vi "Speed Estimation (1 Motor with IC).vi"(0 "waveforms":waveform(dbl)[](array[waveform]), 1 "fundamental frequency [Hz]":dbl=50.0, 2 "reset? (F)":bool, 7 "speed estimation settings":cluster{"% overlap":dbl, "algorithm":T2}={"% overlap"=0.0, "algorithm"=enum."3-phase signals"}, 9 "initial conditions":T1 {"zoom FFT settings"."FFT settings"."window" items=["Rectangle"=0, "Hanning"=1, "Hamming"=2, "Blackman-Harris"=3, "Exact Blackman"=4, "Blackman"=5, "Flat Top"=6, "4 Term B-Harris "=7, "7 Term B-Harris"=8, "Low Sidelobe"=9, "Blackman Nuttall"=11, "Triangle"=30, "Bartlett-Hanning"=31, "Bohman"=32, "Parzen"=33, "Welch"=34, "Kaiser"=60, "Dolph-Chebyshev"=61, "Gaussian"=62]}, 11 "error in (no error)":errorcluster, 12 "nameplate information":T4, 13 "window length (60 s)":dbl=60.0) -> (3 "new data available?":bool, 4 "speed [RPM]":dbl, 6 "slip":dbl, 10 "final conditions":T1 {"zoom FFT settings"."FFT settings"."window" items=["Rectangle"=0, "Hanning"=1, "Hamming"=2, "Blackman-Harris"=3, "Exact Blackman"=4, "Blackman"=5, "Flat Top"=6, "4 Term B-Harris "=7, "7 Term B-Harris"=8, "Low Sidelobe"=9, "Blackman Nuttall"=11, "Triangle"=30, "Bartlett-Hanning"=31, "Bohman"=32, "Parzen"=33, "Welch"=34, "Kaiser"=60, "Dolph-Chebyshev"=61, "Gaussian"=62]}, 15 "error out":errorcluster)   [LabVIEW 2014, in "NI_EP_Motor Monitoring.lvlib"]
doc: "Calculates the motor speed. You must manually select the polymorphic instance you want to use."
uses:
  <vilib>/addons/Electrical Power/Motor Monitoring/NI_EP_Motor Monitoring.lvlib
  <vilib>/addons/Electrical Power/Motor Monitoring/subVIs/ep_Demodulation Algorithm.ctl
  <vilib>/addons/Electrical Power/Motor Monitoring/subVIs/ep_Initial Conditions for Speed Estimation.ctl
  <vilib>/addons/Electrical Power/Motor Monitoring/subVIs/ep_Zoom FFT Settings.ctl
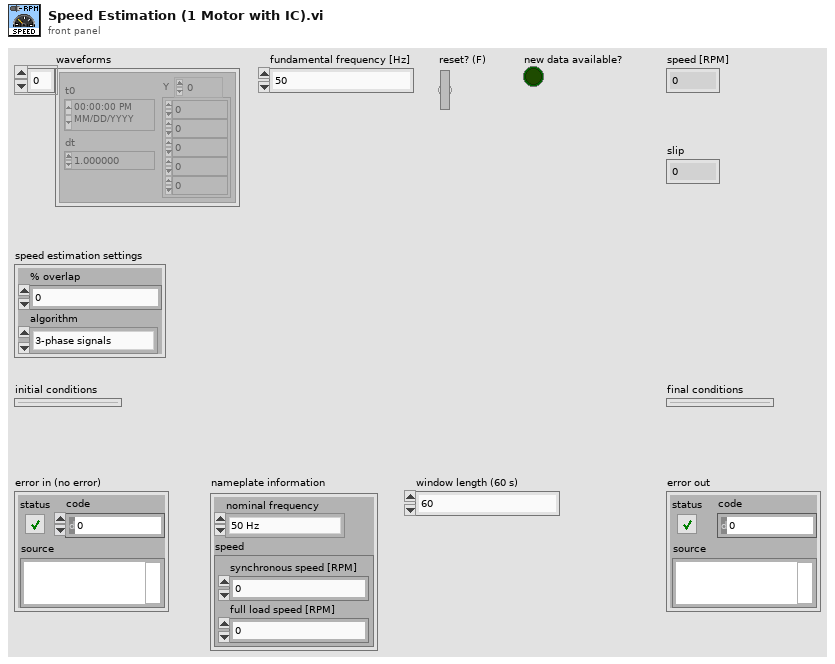
[diagram p1: front panel]
types:
  T1 = typedef "NI_EP_Motor Monitoring.lvlib/ep_Initial Conditions for Speed Estimation.ctl" = cluster{"SVAF state":cluster{"space vector amplitude":dbl, "hilbert state":cluster{"delay conditions":dbl[], "filter conditions":dbl[]}}, "zoom FFT state":cluster{"phase state":dbl, "zoom FFT state":cluster{"zoom settings state":cluster{"zoom":i32, "stop band attenuation":enum16{"84 dB", "96 dB", "120 dB"}, "alias protect in final transition":bool, "oversampling ratio":dbl}, "SML Decimation Filter (complex input) state":cluster{"decimation settings state":cluster{"M":i32, "stop band attenuation":enum16{"84 dB", "96 dB", "120 dB"}, "alias protect in transition band":bool, "oversampling ratio":dbl}, "counter for garbage samples state":i32, "sml_Parameter Setting for Zoom Factor state":cluster{"filter length * interpolation state":i32, "interpolation state":i32, "comb filter order state":i32, "CFIR par state":cluster{"h":dbl[], "M":i32, "N":i32}, "LFIR par state":cluster{"h":dbl[], "M":i32, "N":i32}, "CIC Stages state":i32}, "aal_CIC (complex input) state":cluster{"aal_cascaded moving average (complex input) state":cluster{"states":cdb[], "circular buffers state":cdb[][], "circular buffer counter state":i32}, "aal_moving average with decimation by order (complex input) state":cluster{"residue result state":cdb, "processed data counter state":i32}}, "sml_Cascaded Decimation Filter (complex input) CFIR state":cluster{"unprocessed data state":cdb[], "final conditions state":cdb[][], "sml_M-1 Decimator with IC (complex input) state":cluster{"coefficients in reverse order state":dbl[], "max index for coefficients state":i32}}, "sml_Cascaded Decimation Filter (complex input) LFIR state":cluster{"unprocessed data state":cdb[], "final conditions state":cdb[][], "sml_M-1 Decimator with IC (complex input) state":cluster{"coefficients in reverse order state":dbl[], "max index for coefficients state":i32}}}, "ma_SML Data Packing (complex input) state":cluster{"array getting packed state":cdb[], "last array processed state":cdb[], "index state":i32, "packing parameters state":cluster{i32, "size":i32}}}, "FFT{X} [Vrms]":cdb[]}, "speed state":cluster{"speed [RPM]":dbl, "slip":dbl}, "speed estimation settings":cluster{"% overlap":dbl, "algorithm":T2}, "filter information":cluster{"coefficients":dbl[], "order":i32}, "zoom FFT settings":T3, "last valid window":i32, "fund. frequency for averager":dbl[]}
  T2 = typedef "NI_EP_Motor Monitoring.lvlib/ep_Demodulation Algorithm.ctl" = enum16{"1-phase signal", "3-phase signals"}
  T3 = typedef "NI_EP_Motor Monitoring.lvlib/ep_Zoom FFT Settings.ctl" = cluster{"FFT settings":cluster{"window":u16, "Window Size":i32, "FFT Size":i32, "%overlap":dbl}, "zoom settings":cluster{"zoom":i32, "stop band attenuation":enum16{"84 dB", "96 dB", "120 dB"}, "alias protect in final transition":bool, "oversampling ratio":dbl}, "other settings":cluster{"fmod":dbl, "f0":dbl, "df":dbl, "oidx":i32, "olen":i32}, "iterations":i32, "max block size":i32, "fs":dbl}
  T4 = cluster{"nominal frequency":enum16{"50 Hz", "60 Hz"}, "speed":cluster{"synchronous speed [RPM]":dbl, "full load speed [RPM]":dbl}}
  T5 = cluster{"block size":i32, "window length [s]":dbl, "dt":dbl}
  T6 = cluster{"synchronous speed [RPM]":dbl, "full load speed [RPM]":dbl}
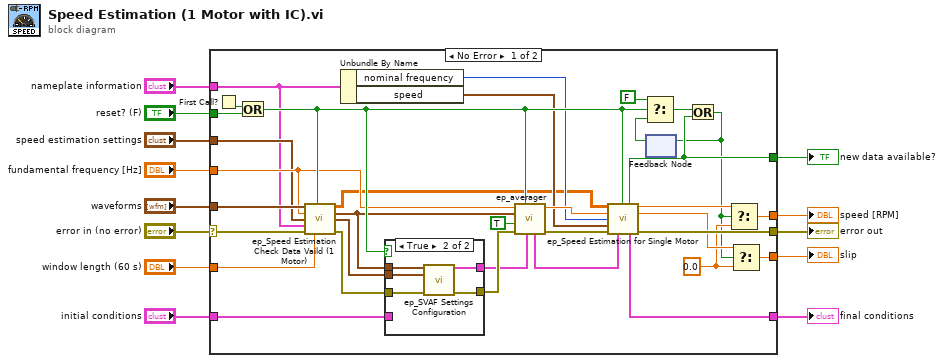
[diagram p0: block diagram]
diagram:
  n1 = case shown="No Error" "error in (no error)" {
    selector: "error in (no error)" -> [w42 w55]
    tunnel: [w44 w55] -> w12
    tunnel: "fundamental frequency [Hz]" -> [w34 _]
    tunnel: "window length (60 s)" -> [w43 _]
    tunnel: "speed estimation settings" -> [w33 _]
    tunnel: "reset? (F)" -> [w46 _]
    tunnel: "waveforms" -> [w45 _]
    tunnel: "nameplate information" -> [w24 _]
    tunnel: [w22 _] -> w6
    tunnel: [w38 _] -> w3
    tunnel: [w28 _] -> w4
    tunnel: [w26 _] -> w1
    tunnel: "initial conditions" -> [w25 _]
    frame No Error {
      w27 = 0.0
      n2 = First Call?() -> (First Call?: T/F=w47:bool)
      n3 = Or(x=w47, y=w46) -> (x .or. y?=w35:bool)
      n4 = call <vilib>:"ep_Speed Estimation Check Data Vaild (1 Motor).vi"("waveforms"=w45, "reset? (F)"=w35, "fundamental frequency [Hz]"=w34, "speed estimation settings"=w33, "nameplate information"=w24, "error in (no error)"=w42, "window length [s]"=w43) -> ("signals"=w23:dbl[][], "spectra parameters"=w17:T5, "dup speed estimation settings"=w30:cluster{"% overlap":dbl, "algorithm":T2}, "error out"=w20:errorcluster)  [unwired: 5 in]
      n5 = Unbundle By Name(w24) -> ("nominal frequency"=w32:enum16{"50 Hz", "60 Hz"}, "speed"=w31:T6)
      n6 = case shown="True" w35 {
        tunnel: w20 -> [w49 w54]
        tunnel: [w49 w53] -> w19
        tunnel: w17 -> [_ w52]
        tunnel: w30 -> [_ w51]
        tunnel: [w48 w50] -> w16
        tunnel: w25 -> [w48 _]
        frame False {
        }
        frame True {
          n7 = call <vilib>:"ep_SVAF Settings Configuration.vi"("spectra parameters"=w52, "speed estimation settings"=w51, "error in (no error)"=w54) -> ("initial conditions"=w50:T1, "error out"=w53:errorcluster)  [unwired: 11 in]
        }
      }
      n8 = call <vilib>:"ep_averager.vi"("initial conditions"=w16, "reset? (F)"=w35, "error in (no error)"=w19, "use initial conditions? (F)"=TRUE, "spectra parameters"=w17, "fundamental frequecy"=w34) -> ("error out"=w18:errorcluster, "average"=w41:dbl, "final conditions"=w15:T1)  [unwired: 3 in]
      n9 = call <vilib>:"ep_Speed Estimation for Single Motor.vi"("signals"=w23, "reset? (F)"=w35, "fundamental frequency [Hz]"=w41, "nominal frequency"=w32, "nameplate speed"=w31, "error in (no error)"=w18, "initial conditions"=w15) -> ("new speed available?"=w22:bool, "speed [RPM]"=w39:dbl, "slip"=w29:dbl, "final conditions"=w26:T1, "error out"=w44:errorcluster)  [unwired: 4 in]
      n10 = feedback #1() -> (w37:bool)  [unwired: 1 in]
      n11 = Select(t=FALSE, s=w35, f=w37) -> (s? t:f=w36:bool)
      n12 = Or(x=w36, y=w22) -> (x .or. y?=w21:bool)
      n13 = feedback-in #1(w21) -> ()
      n14 = Select(t=w39, s=w21, f=w27) -> (s? t:f=w38:dbl)
      n15 = Select(t=w29, s=w21, f=w27) -> (s? t:f=w28:dbl)
    }
    frame Error {
    }
  }
  "error out" <- w12
  "new data available?" <- w6
  "slip" <- w4
  "speed [RPM]" <- w3
  "final conditions" <- w1
